vi "SR830_Keithley_Data_Recorder.vi"() -> ()   [LabVIEW 2021]
uses:
  <instrlib>/Stanford Research 830/Stanford Research 830.lvlib
  <instrlib>/Stanford Research 830/Public/Data/Read (All Parameters).vi
panel:
  out "current time":timestamp
  out "X-Value 3":dbl
  out "Theta-Value 3":dbl
  out "R-Value 3":dbl
  in  "System #3 Enabled/Disabled":bool
  in  "SR830 #3":refnum<visa-resource-name>="GPIB0::10::INSTR"
  in  "SR830 #3 Input Connection":u16(ring) items=["Single-Ended Voltage", "Differential Voltage", "1 MOhm Current Gain", "100 MOhm Current Gain"]
  in  "SR830 #3\nInput Coupling":u16(ring) items=["AC", "DC"]
  in  "SR830 #3 Input \nShield Grounding":u16(ring) items=["Float", "Ground"]
  in  "SR830 #3 Input\nNotch Filter":u16(ring) items=["None", "Line Notch", "2x Line Notch", "Both Notch Filters"]
  in  "SR830 #3 Trigger Source":u16(ring) items=["Internal", "External"]
  in  "SR830 #3 Internal \nReference Frequency":dbl=17.0
  in  "SR830 #3 Detection Harm. Num.":dbl=1.0
  in  "SR830 #3 Sine \nOutput Amplitude":dbl=1.0
  in  "SR830 #3 Reference Source":u16(ring)=1 items=["External", "Internal"]
  in  "SR830 #3 Manual \nPhase":dbl
  in  "SR830 #3 \nAuto Phase":bool
  in  "SR830 #3 \nTime Constant":u16(ring)=9 items=["10 us", "30 us", "100 us", "300 us", "1 ms", "3 ms", "10 ms", "30 ms", "100 ms", "300 ms", "1 s", "3 s", "10 s", "30 s", "100 s", "300 s", "1 ks", "3 ks", "10 ks", "30 ks"]
  in  "SR830 #3 Low\nPass Filter Slope":u16(ring)=3 items=["6 dB/oct", "12 dB/oct", "18 db/oct", "24 dB/oct"]
  in  "SR830 #3\nSync Filter":bool
  in  "SR830 #3 \nDynamic Reserve":i16(ring)=1 items=["Auto Reserve"=-1, "High Reserve"=0, "Normal"=1, "Low Noise"=2]
  in  "SR830 #3\nSensitivity":i16(ring)=17 items=["Auto Gain"=-1, "2 nV/fA"=0, "5 nV/fA"=1, "10 nV/fA"=2, "20 nV/fA"=3, "50 nV/fA"=4, "100 nV/fA"=5, "200 nV/fA"=6, "500 nV/fA"=7, "1 uV/pA"=8, "2 uV/pA"=9, "5 uV/pA"=10, "10 uV/pA"=11, "20 uV/pA"=12, "50 uV/pA"=13, "100 uV/pA"=14, "200 uV/pA"=15, "500 uV/pA"=16, "1 mV/nA"=17, "2 mV/nA"=18, "5 mV/nA"=19, "10 mV/nA"=20, "20 mV/nA"=21, "50 mV/nA"=22, "100 mV/nA"=23, "200 mV/nA"=24, "500 mV/mA"=25, "1 V/uA"=26]
  out "X-Value 2":dbl
  out "Theta-Value 2":dbl
  out "R-Value 2":dbl
  in  "System #2 Enabled/Disabled":bool
  in  "SR830 #2":refnum<visa-resource-name>="GPIB0::10::INSTR"
  in  "SR830 #2 Input Connection":u16(ring) items=["Single-Ended Voltage", "Differential Voltage", "1 MOhm Current Gain", "100 MOhm Current Gain"]
  in  "SR830 #2\nInput Coupling":u16(ring) items=["AC", "DC"]
  in  "SR830 #2 Input \nShield Grounding":u16(ring) items=["Float", "Ground"]
  in  "SR830 #2 Input\nNotch Filter":u16(ring) items=["None", "Line Notch", "2x Line Notch", "Both Notch Filters"]
  in  "SR830 #2 Trigger Source":u16(ring) items=["Internal", "External"]
  in  "SR830 #2 Internal \nReference Frequency":dbl=17.0
  in  "SR830 #2 Detection Harm. Num.":dbl=1.0
  in  "SR830 #2 Sine \nOutput Amplitude":dbl=1.0
  in  "SR830 #2 Reference Source":u16(ring)=1 items=["External", "Internal"]
  in  "SR830 #2 Manual \nPhase":dbl
  in  "SR830 #2 \nAuto Phase":bool
  in  "SR830 #2 \nTime Constant":u16(ring)=9 items=["10 us", "30 us", "100 us", "300 us", "1 ms", "3 ms", "10 ms", "30 ms", "100 ms", "300 ms", "1 s", "3 s", "10 s", "30 s", "100 s", "300 s", "1 ks", "3 ks", "10 ks", "30 ks"]
  in  "SR830 #2 Low\nPass Filter Slope":u16(ring)=3 items=["6 dB/oct", "12 dB/oct", "18 db/oct", "24 dB/oct"]
  in  "SR830 #2\nSync Filter":bool
  in  "SR830 #2 \nDynamic Reserve":i16(ring)=1 items=["Auto Reserve"=-1, "High Reserve"=0, "Normal"=1, "Low Noise"=2]
  in  "SR830 #2\nSensitivity":i16(ring)=17 items=["Auto Gain"=-1, "2 nV/fA"=0, "5 nV/fA"=1, "10 nV/fA"=2, "20 nV/fA"=3, "50 nV/fA"=4, "100 nV/fA"=5, "200 nV/fA"=6, "500 nV/fA"=7, "1 uV/pA"=8, "2 uV/pA"=9, "5 uV/pA"=10, "10 uV/pA"=11, "20 uV/pA"=12, "50 uV/pA"=13, "100 uV/pA"=14, "200 uV/pA"=15, "500 uV/pA"=16, "1 mV/nA"=17, "2 mV/nA"=18, "5 mV/nA"=19, "10 mV/nA"=20, "20 mV/nA"=21, "50 mV/nA"=22, "100 mV/nA"=23, "200 mV/nA"=24, "500 mV/mA"=25, "1 V/uA"=26]
  out "R-Value":dbl
  out "Theta-Value":dbl
  out "X-Value":dbl
  in  "SR830 #1\nSensitivity":i16(ring)=17 items=["Auto Gain"=-1, "2 nV/fA"=0, "5 nV/fA"=1, "10 nV/fA"=2, "20 nV/fA"=3, "50 nV/fA"=4, "100 nV/fA"=5, "200 nV/fA"=6, "500 nV/fA"=7, "1 uV/pA"=8, "2 uV/pA"=9, "5 uV/pA"=10, "10 uV/pA"=11, "20 uV/pA"=12, "50 uV/pA"=13, "100 uV/pA"=14, "200 uV/pA"=15, "500 uV/pA"=16, "1 mV/nA"=17, "2 mV/nA"=18, "5 mV/nA"=19, "10 mV/nA"=20, "20 mV/nA"=21, "50 mV/nA"=22, "100 mV/nA"=23, "200 mV/nA"=24, "500 mV/mA"=25, "1 V/uA"=26]
  in  "SR830 #1 \nDynamic Reserve":i16(ring)=1 items=["Auto Reserve"=-1, "High Reserve"=0, "Normal"=1, "Low Noise"=2]
  in  "SR830 #1\nSync Filter":bool
  in  "SR830 #1 Low\nPass Filter Slope":u16(ring)=3 items=["6 dB/oct", "12 dB/oct", "18 db/oct", "24 dB/oct"]
  in  "SR830 #1 \nTime Constant":u16(ring)=8 items=["10 us", "30 us", "100 us", "300 us", "1 ms", "3 ms", "10 ms", "30 ms", "100 ms", "300 ms", "1 s", "3 s", "10 s", "30 s", "100 s", "300 s", "1 ks", "3 ks", "10 ks", "30 ks"]
  in  "SR830 #1 \nAuto Phase":bool
  in  "SR830 #1 Manual \nPhase":dbl
  in  "SR830 #1 Reference Source":u16(ring)=1 items=["External", "Internal"]
  in  "SR830 #1 Sine \nOutput Amplitude":dbl=1.0
  in  "SR830 #1 Detection Harm. Num.":dbl=1.0
  in  "SR830 #1 Internal \nReference Frequency":dbl=17.0
  in  "SR830 #1 Trigger Source":u16(ring) items=["Internal", "External"]
  in  "SR830 #1 Input\nNotch Filter":u16(ring) items=["None", "Line Notch", "2x Line Notch", "Both Notch Filters"]
  in  "SR830 #1 Input \nShield Grounding":u16(ring) items=["Float", "Ground"]
  in  "SR830 #1\nInput Coupling":u16(ring) items=["AC", "DC"]
  in  "SR830 #1 Input Connection":u16(ring) items=["Single-Ended Voltage", "Differential Voltage", "1 MOhm Current Gain", "100 MOhm Current Gain"]
  in  "SR830 #1":refnum<visa-resource-name>="GPIB0::10::INSTR"
  in  "System #1 Enabled/Disabled":bool
  in  "System Reset All?":bool
  in  "program_stop":bool
  out "Actual Save Path":path
  in  "<File Name>.txt (Don't add extension)":string
  in  "Data Save Path:":path=path "C:/Users/labpc/Documents/ProbeStation Users Data"
  # "SR830"
  # "SR830"
  # "SR830"
  # "Input Signal"
  # "Input Signal"
  # "Input Signal"
  # "Readout (Recorded)"
  # "Readout (Recorded)"
  # "Readout (Recorded)"
  # "Source / Reference"
  # "Source / Reference"
  # "Source / Reference"
  # "Input Filters & Sens"
  # "Input Filters & Sens"
  # "Input Filters & Sens"
  # "Initialisation:\n--> Reset \n--> Instruments?"
  # "File I/O"
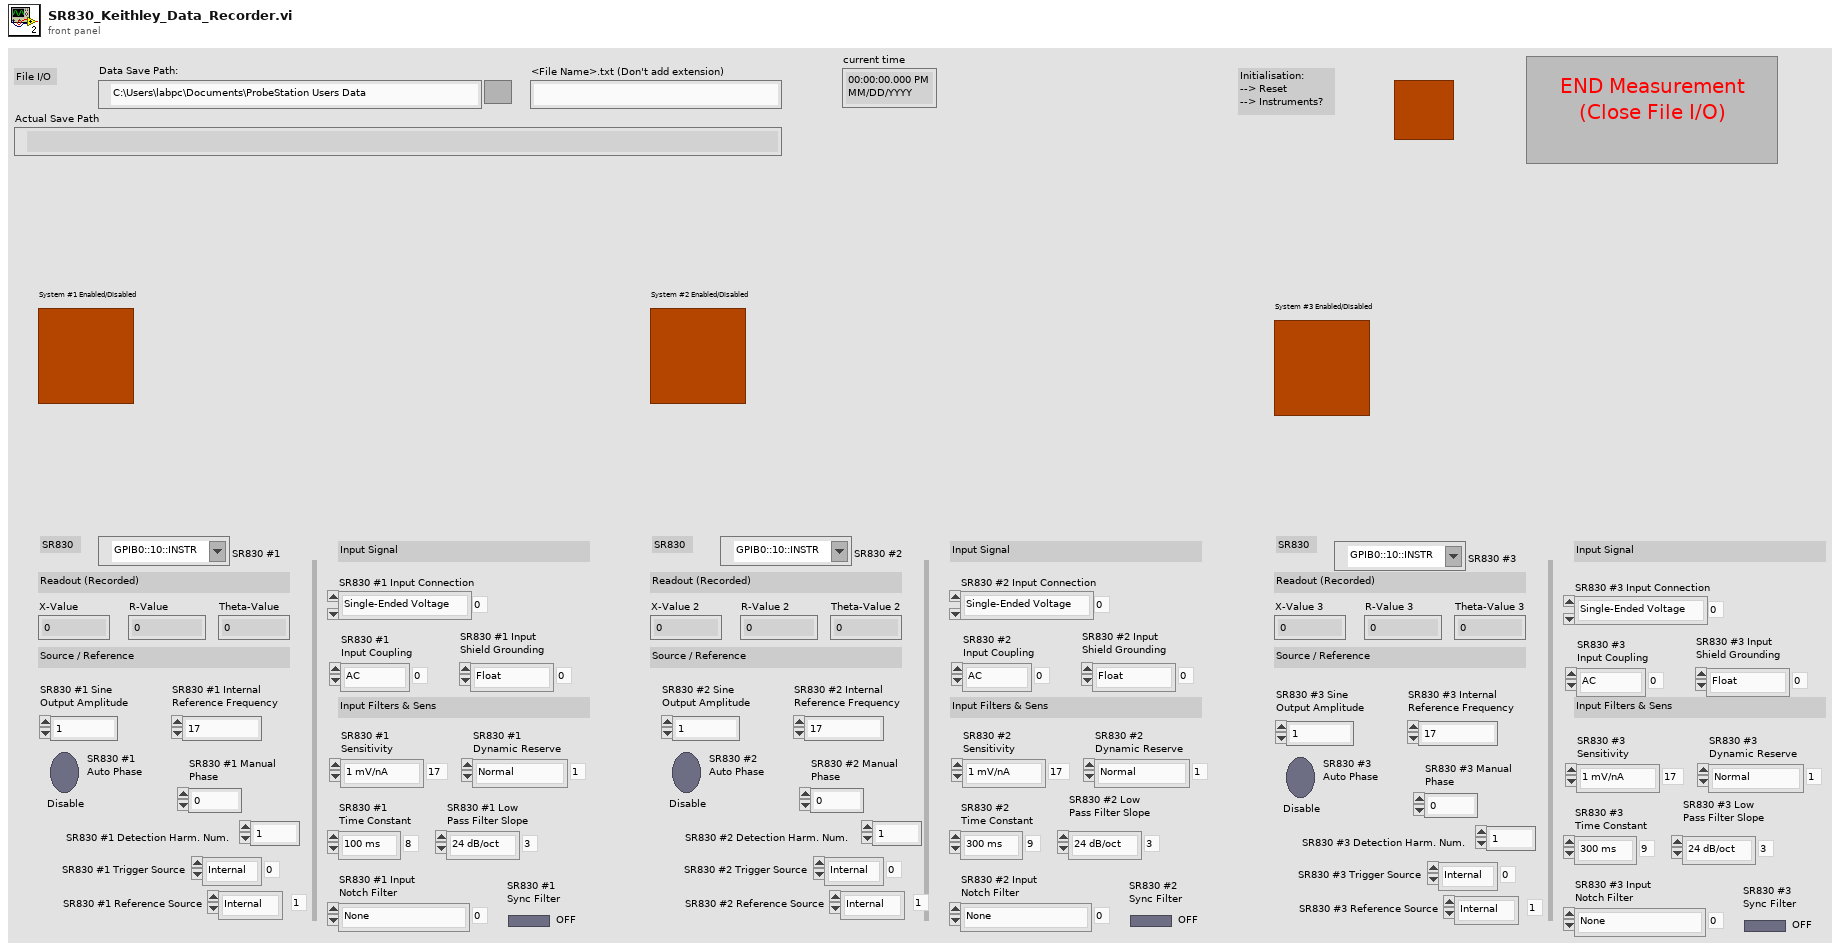
[diagram p1: front panel]
types:
  T1 = enum16{"open", "replace", "create", "open or create", "replace or create", "replace or create with confirmation"}
  T2 = cluster{"VISA resource name out":refnum<visa-resource-name>, "error out":errorcluster}
  T3 = cluster{"array":dbl[][], "array":dbl[][], "array":dbl[][]}
  T4 = cluster{"System #1 Enabled/Disabled":bool, "System #2 Enabled/Disabled":bool, "System #3 Enabled/Disabled":bool}
  T5 = cluster{"Voltage":sgl, "Current":sgl, "X-Value":dbl}
  T6 = cluster{"X-Value":dbl, "Y-Value":dbl, "R-Value":dbl, "Theta-Value":dbl, "Aux In 1 Value":dbl, "Aux In 2 Value":dbl, "Aux In 3 Value":dbl, "Aux In 4 Value":dbl, "Reference Frequency":dbl, "Channel 1 Display":dbl, "Channel 2 Display":dbl}
  T7 = cluster{"X-Value":dbl, "R-Value":dbl, "Theta-Value":dbl}
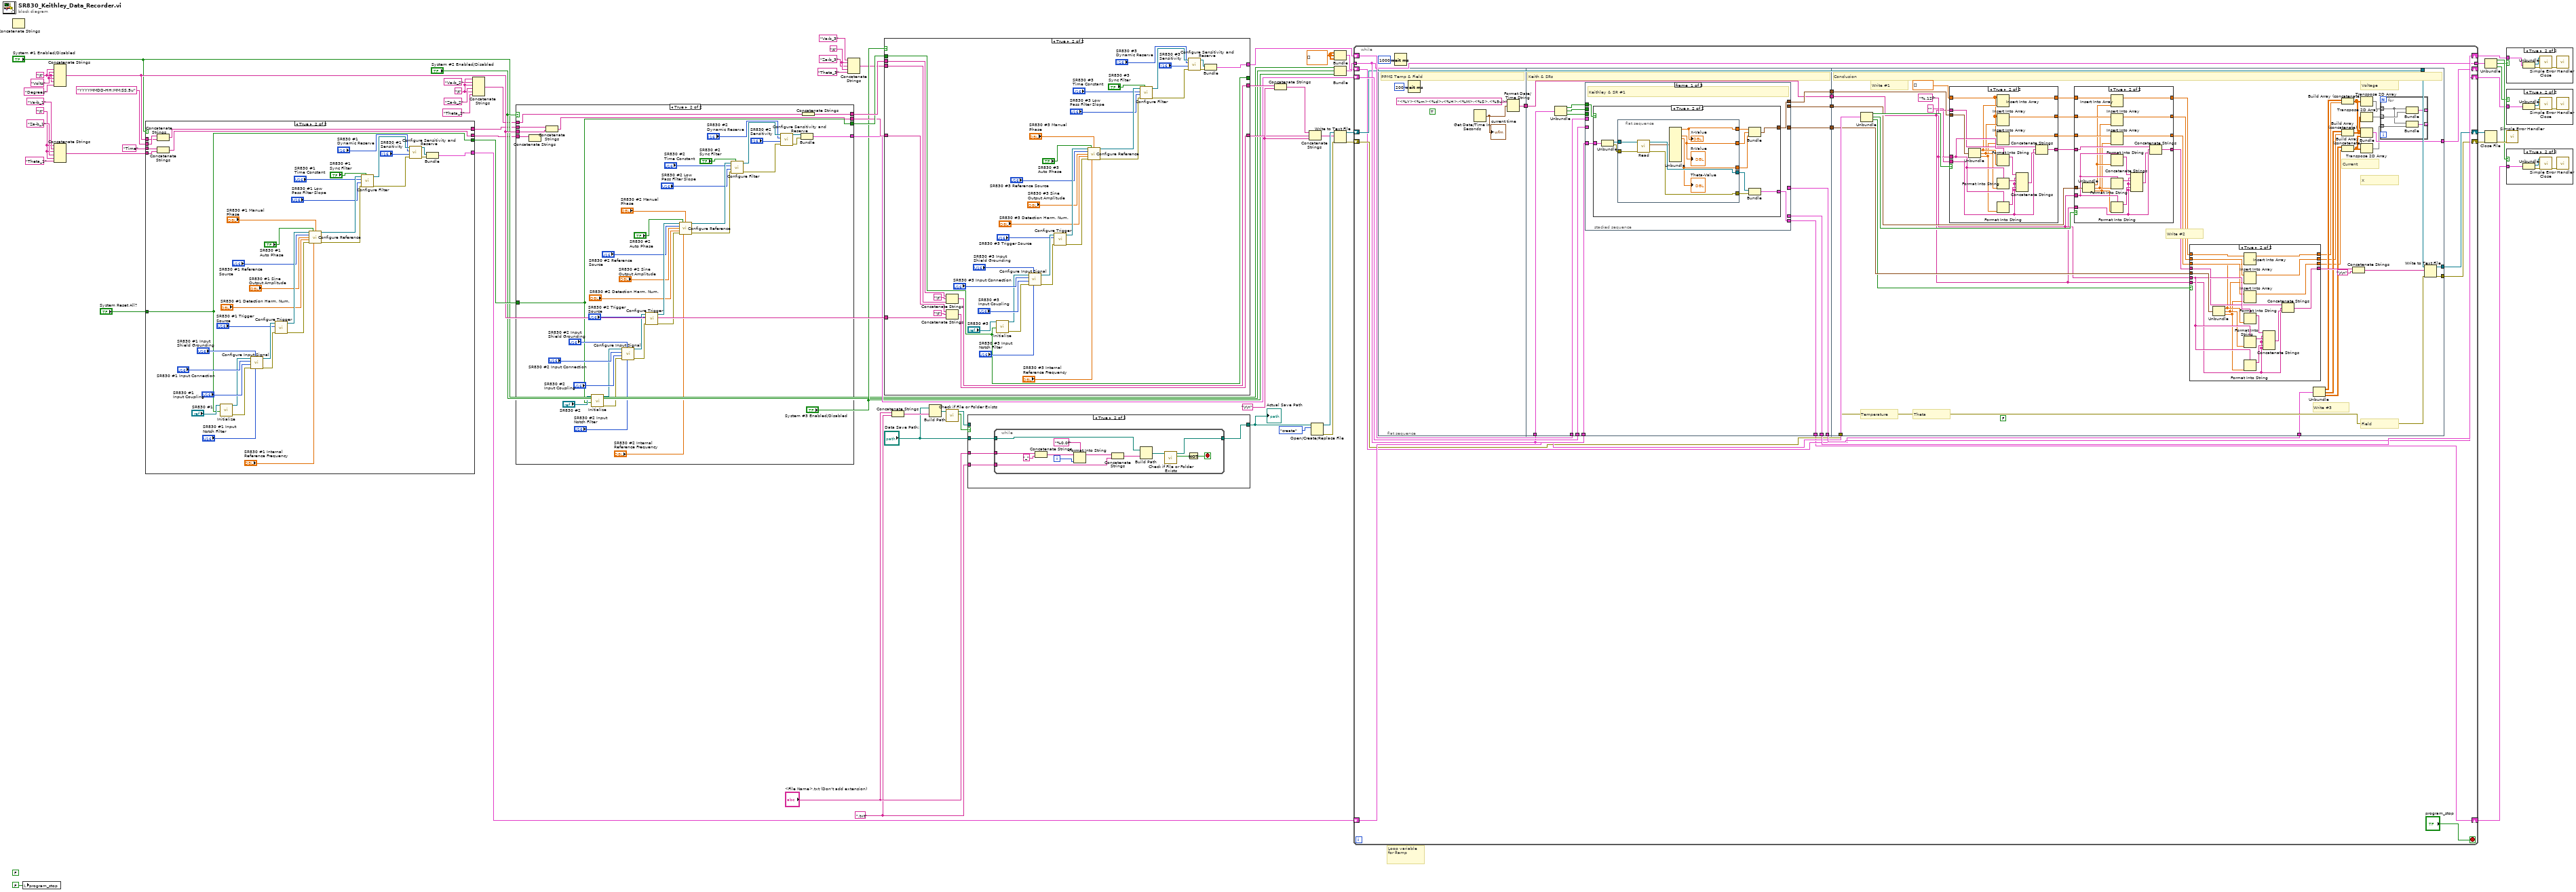
[diagram p0: block diagram]
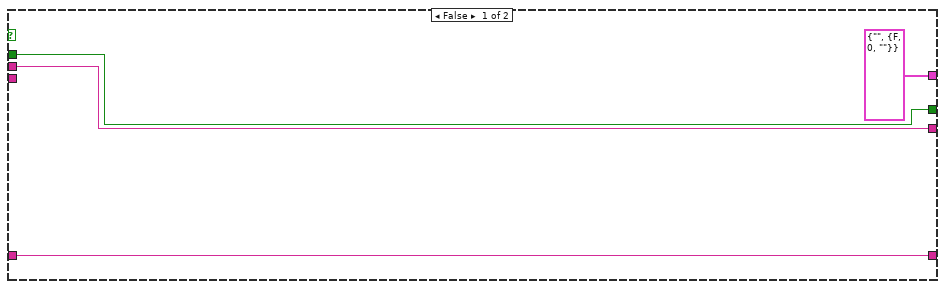
[diagram p5: hidden frame]
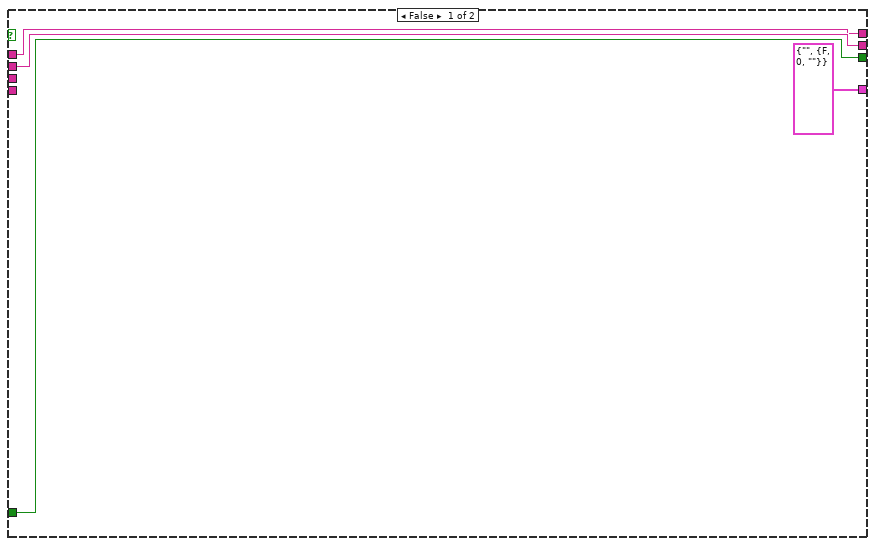
[diagram p6: hidden frame]
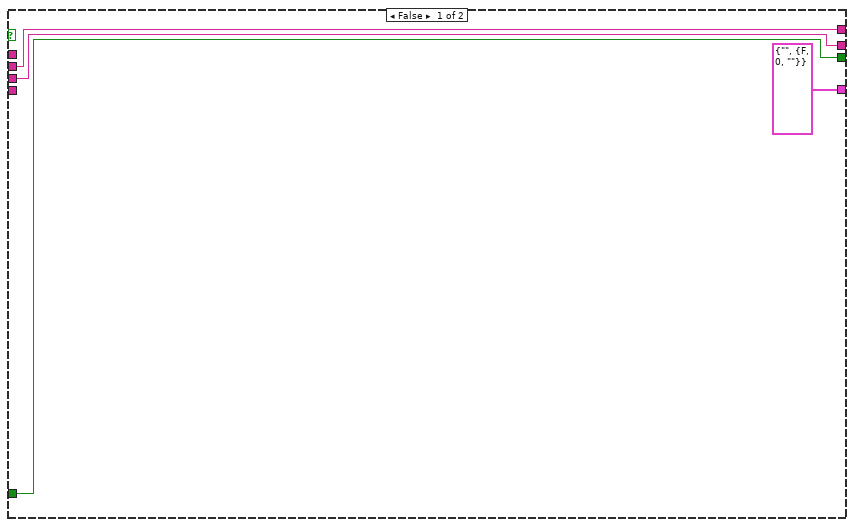
[diagram p7: hidden frame]
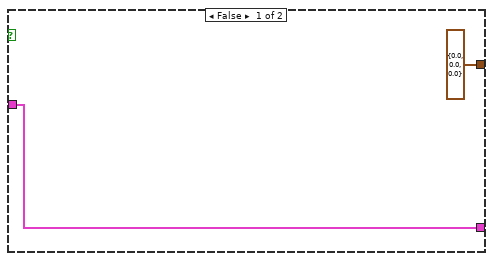
[diagram p9: hidden frame]
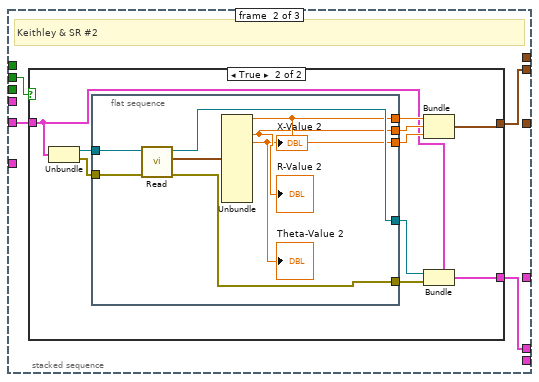
[diagram p10: hidden frame]
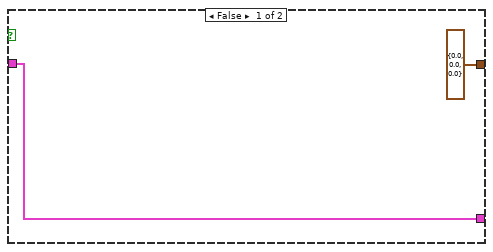
[diagram p11: hidden frame]
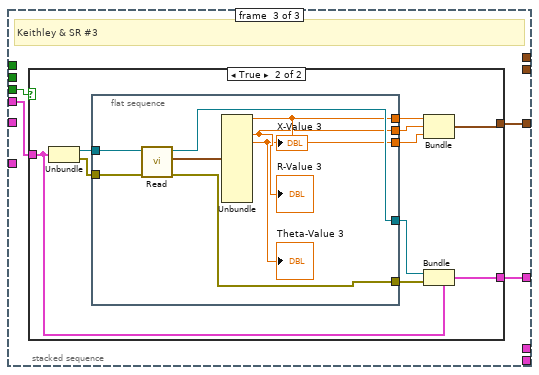
[diagram p12: hidden frame]
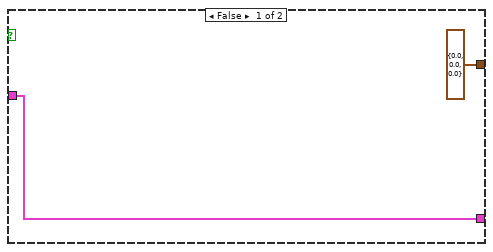
[diagram p13: hidden frame]
diagram:
  w15 = "\t"
  w3 = "\t"
  w26 = dbl[][] [] ("array")
  w4 = "\t"
  w6 = "Volts" ("string")
  w47 = "\r\n"
  w8 = "\t"
  w60 = ".txt"
  (unwired) FALSE ("Measuring")
  # "Loop variable \nfor Ramp"
  n1 = Concatenate Strings() -> ()  [unwired: 3 in, 1 out]
  n2 = local write "program_stop"(FALSE ("program_stop")) -> ()
  n3 = Concatenate Strings(w4, w6, w4, w6, w4, "Degrees" ("string")) -> (w50:string)  [unwired: 1 in]
  n4 = Concatenate Strings(w8, "Va-b_1" ("string"), w8, "Za-b_1" ("string"), w8, "Theta_1" ("string")) -> (w54:string)
  n5 = case shown="True" "System #1 Enabled/Disabled" {
    tunnel: w54 -> [_ w73]
    tunnel: "System Reset All?" -> [w70 w80]
    tunnel: [w70 w80] -> w56
    tunnel: [w68 w79] -> w2
    tunnel: w50 -> [_ w72]
    tunnel: [T2 {"VISA resource name out"="", "error out"={"status"=FALSE, "code"=0, "source"=""}} w76] -> w39
    tunnel: "Time" ("string") -> [w68 w75]
    tunnel: "YYYYMMDD-HH:MM:SS.5u" ("string") -> [w67 w74]
    tunnel: [w67 w71] -> w1
    frame False {
    }
    frame True {
      n6 = Concatenate Strings(w74, w72) -> (w71:string)
      n7 = Concatenate Strings(w75, w73) -> (w79:string)
      n8 = call <instrlib>:"Initialize.vi"("Reset (True)"=w80, "VISA resource name"="SR830 #1") -> ("error out"=w103:errorcluster, "VISA resource name out"=w104:refnum<visa-resource-name>)  [unwired: 8 in]
      n9 = call <instrlib>:"Configure Input Signal.vi"("Input Notch Filter (0: None)"="SR830 #1 Input\nNotch Filter", "Input Shield Grounding (0: Float)"="SR830 #1 Input \nShield Grounding", "error in (no error)"=w103, "Input Coupling (0: AC)"="SR830 #1\nInput Coupling", "Input Connection (0: Single-Ended Voltage)"="SR830 #1 Input Connection", "VISA resource name"=w104) -> ("error out"=w101:errorcluster, "VISA resource name out"=w102:refnum<visa-resource-name>)  [unwired: 4 in]
      n10 = call <instrlib>:"Configure Trigger.vi"("error in (no error)"=w101, "Trigger Source (0: Internal)"="SR830 #1 Trigger Source", "VISA resource name"=w102) -> ("error out"=w99:errorcluster, "VISA resource name out"=w100:refnum<visa-resource-name>)  [unwired: 7 in]
      n11 = call <instrlib>:"Configure Reference.vi"("VISA resource name"=w100, "Auto Phase (T: Enabled)"="SR830 #1 \nAuto Phase", "Manual Phase (0 Degree)"="SR830 #1 Manual \nPhase", "Reference Source (1: Internal)"="SR830 #1 Reference Source", "Sine Output Amplitude (1 V)"="SR830 #1 Sine \nOutput Amplitude", "Detection Harmonic Number (1)"="SR830 #1 Detection Harm. Num.", "error in (no error)"=w99, "Internal Reference Frequency (1000 Hz)"="SR830 #1 Internal \nReference Frequency") -> ("VISA resource name out"=w97:refnum<visa-resource-name>, "error out"=w98:errorcluster)  [unwired: 6 in]
      n12 = call <instrlib>:"Configure Filter.vi"("Enable Sync Filter (F: Disable)"="SR830 #1\nSync Filter", "error in (no error)"=w98, "Low Pass Filter Slope (1: 12dB/oct)"="SR830 #1 Low\nPass Filter Slope", "Time Constant (8: 100ms)"="SR830 #1 \nTime Constant", "VISA resource name"=w97) -> ("error out"=w83:errorcluster, "VISA resource name out"=w84:refnum<visa-resource-name>)  [unwired: 5 in]
      n13 = call <instrlib>:"Configure Sensitivity and Reserve.vi"("error in (no error)"=w83, "Sensitivity (-1: Auto gain)"="SR830 #1\nSensitivity", "Dynamic Reserve (-1: Auto Reserve)"="SR830 #1 \nDynamic Reserve", "VISA resource name"=w84) -> ("error out"=w77:errorcluster, "VISA resource name out"=w78:refnum<visa-resource-name>)  [unwired: 6 in]
      n14 = Bundle("VISA resource name out"=w78, "error out"=w77) -> (w76:T2)  [unwired: 1 in]
    }
  }
  n15 = Concatenate Strings(w3, "Va-b_2" ("string"), w3, "Za-b_2" ("string"), w3, "Theta_2" ("string")) -> (w11:string)
  n16 = case shown="True" "System #2 Enabled/Disabled" {
    tunnel: w11 -> [w108 w148]
    tunnel: [w108 w147] -> w55
    tunnel: w56 -> [w111 w119]
    tunnel: [w111 w119] -> w53
    tunnel: w1 -> [w110 w118]
    tunnel: [w110 w117] -> w51
    tunnel: w50 -> [_ w112]
    tunnel: [T2 {"VISA resource name out"="", "error out"={"status"=FALSE, "code"=0, "source"=""}} w114] -> w38
    tunnel: w2 -> [_ w113]
    frame False {
    }
    frame True {
      n17 = Concatenate Strings(w113) -> ()  [unwired: 1 in, 1 out]
      n18 = Concatenate Strings(w118, w112) -> (w117:string)
      n19 = call <instrlib>:"Initialize.vi"("Reset (True)"=w119, "VISA resource name"="SR830 #2") -> ("error out"=w142:errorcluster, "VISA resource name out"=w143:refnum<visa-resource-name>)  [unwired: 8 in]
      n20 = call <instrlib>:"Configure Input Signal.vi"("Input Notch Filter (0: None)"="SR830 #2 Input\nNotch Filter", "Input Shield Grounding (0: Float)"="SR830 #2 Input \nShield Grounding", "error in (no error)"=w142, "Input Coupling (0: AC)"="SR830 #2\nInput Coupling", "Input Connection (0: Single-Ended Voltage)"="SR830 #2 Input Connection", "VISA resource name"=w143) -> ("error out"=w140:errorcluster, "VISA resource name out"=w141:refnum<visa-resource-name>)  [unwired: 4 in]
      n21 = call <instrlib>:"Configure Trigger.vi"("error in (no error)"=w140, "Trigger Source (0: Internal)"="SR830 #2 Trigger Source", "VISA resource name"=w141) -> ("error out"=w138:errorcluster, "VISA resource name out"=w139:refnum<visa-resource-name>)  [unwired: 7 in]
      n22 = call <instrlib>:"Configure Reference.vi"("VISA resource name"=w139, "Auto Phase (T: Enabled)"="SR830 #2 \nAuto Phase", "Manual Phase (0 Degree)"="SR830 #2 Manual \nPhase", "Reference Source (1: Internal)"="SR830 #2 Reference Source", "Sine Output Amplitude (1 V)"="SR830 #2 Sine \nOutput Amplitude", "Detection Harmonic Number (1)"="SR830 #2 Detection Harm. Num.", "error in (no error)"=w138, "Internal Reference Frequency (1000 Hz)"="SR830 #2 Internal \nReference Frequency") -> ("VISA resource name out"=w136:refnum<visa-resource-name>, "error out"=w137:errorcluster)  [unwired: 6 in]
      n23 = call <instrlib>:"Configure Filter.vi"("Enable Sync Filter (F: Disable)"="SR830 #2\nSync Filter", "error in (no error)"=w137, "Low Pass Filter Slope (1: 12dB/oct)"="SR830 #2 Low\nPass Filter Slope", "Time Constant (8: 100ms)"="SR830 #2 \nTime Constant", "VISA resource name"=w136) -> ("error out"=w122:errorcluster, "VISA resource name out"=w123:refnum<visa-resource-name>)  [unwired: 5 in]
      n24 = call <instrlib>:"Configure Sensitivity and Reserve.vi"("error in (no error)"=w122, "Sensitivity (-1: Auto gain)"="SR830 #2\nSensitivity", "Dynamic Reserve (-1: Auto Reserve)"="SR830 #2 \nDynamic Reserve", "VISA resource name"=w123) -> ("error out"=w115:errorcluster, "VISA resource name out"=w116:refnum<visa-resource-name>)  [unwired: 6 in]
      n25 = Bundle("VISA resource name out"=w116, "error out"=w115) -> (w114:T2)  [unwired: 1 in]
      n26 = Concatenate Strings(w148) -> (w147:string)
    }
  }
  n27 = Concatenate Strings("Va-b_3" ("string"), w15, "Za-b_3" ("string"), w15, "Theta_3" ("string")) -> (w10:string)
  n28 = case shown="True" "System #3 Enabled/Disabled" {
    tunnel: w10 -> [_ w191]
    tunnel: w55 -> [w152 w189]
    tunnel: [w152 w188] -> w52
    tunnel: w53 -> [w151 w160]
    tunnel: [w151 w160] -> _
    tunnel: w51 -> [w150 w158]
    tunnel: w50 -> [_ w157]
    tunnel: [w150 w156] -> w45
    tunnel: [T2 {"VISA resource name out"="", "error out"={"status"=FALSE, "code"=0, "source"=""}} w153] -> w37
    frame False {
    }
    frame True {
      n29 = Concatenate Strings(w189, "\t", w191) -> (w188:string)
      n30 = Concatenate Strings(w158, "\t", w157) -> (w156:string)
      n31 = call <instrlib>:"Initialize.vi"("Reset (True)"=w160, "VISA resource name"="SR830 #3") -> ("error out"=w183:errorcluster, "VISA resource name out"=w184:refnum<visa-resource-name>)  [unwired: 8 in]
      n32 = call <instrlib>:"Configure Input Signal.vi"("Input Notch Filter (0: None)"="SR830 #3 Input\nNotch Filter", "Input Shield Grounding (0: Float)"="SR830 #3 Input \nShield Grounding", "error in (no error)"=w183, "Input Coupling (0: AC)"="SR830 #3\nInput Coupling", "Input Connection (0: Single-Ended Voltage)"="SR830 #3 Input Connection", "VISA resource name"=w184) -> ("error out"=w181:errorcluster, "VISA resource name out"=w182:refnum<visa-resource-name>)  [unwired: 4 in]
      n33 = call <instrlib>:"Configure Trigger.vi"("error in (no error)"=w181, "Trigger Source (0: Internal)"="SR830 #3 Trigger Source", "VISA resource name"=w182) -> ("error out"=w179:errorcluster, "VISA resource name out"=w180:refnum<visa-resource-name>)  [unwired: 7 in]
      n34 = call <instrlib>:"Configure Reference.vi"("VISA resource name"=w180, "Auto Phase (T: Enabled)"="SR830 #3 \nAuto Phase", "Manual Phase (0 Degree)"="SR830 #3 Manual \nPhase", "Reference Source (1: Internal)"="SR830 #3 Reference Source", "Sine Output Amplitude (1 V)"="SR830 #3 Sine \nOutput Amplitude", "Detection Harmonic Number (1)"="SR830 #3 Detection Harm. Num.", "error in (no error)"=w179, "Internal Reference Frequency (1000 Hz)"="SR830 #3 Internal \nReference Frequency") -> ("VISA resource name out"=w177:refnum<visa-resource-name>, "error out"=w178:errorcluster)  [unwired: 6 in]
      n35 = call <instrlib>:"Configure Filter.vi"("Enable Sync Filter (F: Disable)"="SR830 #3\nSync Filter", "error in (no error)"=w178, "Low Pass Filter Slope (1: 12dB/oct)"="SR830 #3 Low\nPass Filter Slope", "Time Constant (8: 100ms)"="SR830 #3 \nTime Constant", "VISA resource name"=w177) -> ("error out"=w163:errorcluster, "VISA resource name out"=w164:refnum<visa-resource-name>)  [unwired: 5 in]
      n36 = call <instrlib>:"Configure Sensitivity and Reserve.vi"("error in (no error)"=w163, "Sensitivity (-1: Auto gain)"="SR830 #3\nSensitivity", "Dynamic Reserve (-1: Auto Reserve)"="SR830 #3 \nDynamic Reserve", "VISA resource name"=w164) -> ("error out"=w154:errorcluster, "VISA resource name out"=w155:refnum<visa-resource-name>)  [unwired: 6 in]
      n37 = Bundle("VISA resource name out"=w155, "error out"=w154) -> (w153:T2)  [unwired: 1 in]
    }
  }
  n38 = Concatenate Strings("<File Name>.txt (Don't add extension)", w60) -> (w66:string)
  n39 = Build Path(base path="Data Save Path:", name or relative path=w66) -> (appended path=w65:path)
  n40 = call <vilib>:"Check if File or Folder Exists.vi"("path"=w65) -> ("file or folder exists?"=w64:bool, "dup path"=w63:path)  [unwired: 8 in, 1 out]
  n41 = case shown="True" w64 {
    tunnel: [w192 w193] -> w58
    tunnel: w63 -> [w192 _]
    tunnel: "Data Save Path:" -> [_ w194]
    tunnel: "<File Name>.txt (Don't add extension)" -> [_ w196]
    tunnel: w60 -> [_ w195]
    frame False {
    }
    frame True {
      n42 = while {
        tunnel: w196 -> [w199]
        tunnel: w195 -> [w204]
        tunnel: w194 -> [w202]
        tunnel: [w200] -> w193
        i -> [w206]
        stop <- w208 stop-if-true
        n43 = Concatenate Strings(w199, "_" ("string")) -> (w198:string)
        n44 = Format Into String(format string="%0.0f", initial string=w198, w206) -> (resulting string=w205:string)  [unwired: 1 in, 1 out]
        n45 = Concatenate Strings(w205, w204) -> (w203:string)
        n46 = Build Path(base path=w202, name or relative path=w203) -> (appended path=w201:path)
        n47 = call <vilib>:"Check if File or Folder Exists.vi"("path"=w201) -> ("file or folder exists?"=w209:bool, "dup path"=w200:path)  [unwired: 8 in, 1 out]
        n48 = Not(x=w209) -> (.not. x?=w208:bool)
      }
    }
  }
  "Actual Save Path" <- w58
  n49 = Concatenate Strings(w52, w47) -> (w46:string)
  n50 = Concatenate Strings(w46, w45, w47) -> (w44:string)
  n51 = Open/Create/Replace File(file path (use dialog)=w58, operation (0:open)=T1."create") -> (refnum out=w49:refnum<file>, error out=w48:errorcluster)  [unwired: 4 in, 1 out]
  n52 = Bundle("array"=w26, "array"=w26, "array"=w26) -> (w27:T3)  [unwired: 1 in]
  n53 = Bundle("System #1 Enabled/Disabled"="System #1 Enabled/Disabled", "System #2 Enabled/Disabled"="System #2 Enabled/Disabled", "System #3 Enabled/Disabled"="System #3 Enabled/Disabled") -> (w33:T4)  [unwired: 1 in]
  n54 = Write to Text File(file (use dialog)=w49, text=w44, error in=w48) -> (refnum out=w28:refnum<file>, error out=w42:errorcluster)  [unwired: 1 in, 1 out]
  n55 = while {
    shift-right: [w217] -> w41
    shift-left: w28 -> [w218]
    shift-right: [w215] -> w40
    shift-left: w42 -> [w216]
    shift-right: [w213] -> w25
    shift-left: w39 -> [w227]
    shift-right: [w224] -> w23
    shift-left: w38 -> [w226]
    shift-right: [w223] -> w24
    shift-left: w37 -> [w225]
    tunnel: w33 -> [w219]
    tunnel: [w219] -> w32
    shift-right: [w212] -> _
    shift-left: w27 -> [w214]
    stop <- "program_stop" stop-if-true
    n56 = flat-sequence {
      tunnel: [w230] -> w211
      tunnel: w227 -> [w238]
      tunnel: w226 -> [w247]
      tunnel: w225 -> [w246]
      tunnel: [w236] -> w224
      tunnel: [w235] -> w223
      tunnel: w219 -> [w245]
      tunnel: [w241] -> w222
      tunnel: [w240] -> w221
      tunnel: [w239] -> w220
      tunnel: [w237] -> w213
      tunnel: w211 -> [w234]
      tunnel: [w234] -> w210
      tunnel: w222 -> [w357]
      tunnel: w221 -> [w356]
      tunnel: w220 -> [w355]
      tunnel: w219 -> [w359]
      tunnel: w218 -> [w346]
      tunnel: w216 -> [w344]
      tunnel: [w345] -> w217
      tunnel: [w343] -> w215
      tunnel: w214 -> [w339]
      tunnel: [w338] -> w212
      tunnel: w210 -> [w321]
      frame #0 {
        (unwired) TRUE ("Measuring")
        # "PPMS Temp & Field"
        n57 = Wait (ms)(milliseconds to wait=u32 200) -> ()  [unwired: 1 out]
        n58 = Get Date/Time In Seconds() -> (seconds since 1Jan1904=w232:timestamp)
        "current time" <- w232
        n59 = Format Date/Time String(time format string (%c)="<%Y><%m><%d>-<%H>:<%M>:<%S>.<%5u>" ("string"), seconds (now)=w232) -> (date/time string=w230:string)  [unwired: 1 in]
      }
      frame #1 {
        # "Keith & SRs"
        n60 = Unbundle(w245) -> ("System #1 Enabled/Disabled"=w244:bool, "System #2 Enabled/Disabled"=w243:bool, "System #3 Enabled/Disabled"=w242:bool)
        n61 = stacked-sequence {
          tunnel: w247 -> [_ w275 _]
          tunnel: w246 -> [_ _ w299]
          tunnel: [w248 _ _] -> w237
          tunnel: [_ w272 _] -> w236
          tunnel: w244 -> [w251 _ _]
          tunnel: w243 -> [_ w274 _]
          tunnel: w242 -> [_ _ w298]
          tunnel: [w250 _ _] -> w241
          tunnel: [_ w273 _] -> w240
          tunnel: [_ _ w297] -> w239
          tunnel: w238 -> [w249 _ _]
          tunnel: [_ _ w296] -> w235
          frame #0 {
            # "Keithley & SR #1"
            n62 = case shown="True" w251 {
              tunnel: [w252 w263] -> w248
              tunnel: [T5 {"Voltage"=0.0, "Current"=0.0, "X-Value"=0.0} w257] -> w250
              tunnel: w249 -> [w252 w256]
              frame False {
              }
              frame True {
                n63 = Unbundle(w256) -> ("VISA resource name out"=w255:refnum<visa-resource-name>, "error out"=w254:errorcluster)
                n64 = flat-sequence {
                  tunnel: [w271] -> w262
                  tunnel: [w270] -> w261
                  tunnel: [w268] -> w260
                  tunnel: [w267] -> w259
                  tunnel: [w266] -> w258
                  tunnel: w255 -> [w265]
                  tunnel: w254 -> [w264]
                  frame #0 {
                    n65 = call-poly <instrlib>:"Read.vi"("error in (no error)"=w264, "VISA resource name"=w265) -> ("error out"=w270:errorcluster, "Parameter Values"=w269:T6, "VISA resource name out"=w271:refnum<visa-resource-name>)  [unwired: 7 in]
                    n66 = Unbundle(w269) -> ("X-Value"=w268:dbl, "R-Value"=w267:dbl, "Theta-Value"=w266:dbl)  [unwired: 8 out]
                    "X-Value" <- w268
                    "Theta-Value" <- w266
                    "R-Value" <- w267
                  }
                }
                n67 = Bundle("X-Value"=w260, "R-Value"=w259, "Theta-Value"=w258) -> (w257:T7)  [unwired: 1 in]
                n68 = Bundle("VISA resource name out"=w262, "error out"=w261) -> (w263:T2)  [unwired: 1 in]
              }
            }
          }
          frame #1 {
            # "Keithley & SR #2"
            n69 = case shown="True" w274 {
              tunnel: [w277 w287] -> w272
              tunnel: w275 -> [w277 w283]
              tunnel: [T5 {"Voltage"=0.0, "Current"=0.0, "X-Value"=0.0} w282] -> w273
              frame False {
              }
              frame True {
                n70 = Unbundle(w283) -> ("VISA resource name out"=w281:refnum<visa-resource-name>, "error out"=w280:errorcluster)
                n71 = flat-sequence {
                  tunnel: [w295] -> w279
                  tunnel: [w294] -> w278
                  tunnel: [w292] -> w286
                  tunnel: [w291] -> w285
                  tunnel: [w290] -> w284
                  tunnel: w281 -> [w289]
                  tunnel: w280 -> [w288]
                  frame #0 {
                    n72 = call-poly <instrlib>:"Read.vi"("error in (no error)"=w288, "VISA resource name"=w289) -> ("error out"=w294:errorcluster, "Parameter Values"=w293:T6, "VISA resource name out"=w295:refnum<visa-resource-name>)  [unwired: 7 in]
                    n73 = Unbundle(w293) -> ("X-Value"=w292:dbl, "R-Value"=w291:dbl, "Theta-Value"=w290:dbl)  [unwired: 8 out]
                    "X-Value 2" <- w292
                    "Theta-Value 2" <- w290
                    "R-Value 2" <- w291
                  }
                }
                n74 = Bundle("X-Value"=w286, "R-Value"=w285, "Theta-Value"=w284) -> (w282:T7)  [unwired: 1 in]
                n75 = Bundle(cluster=w283, "VISA resource name out"=w279, "error out"=w278) -> (w287:T2)
              }
            }
          }
          frame #2 {
            # "Keithley & SR #3"
            n76 = case shown="True" w298 {
              tunnel: [w301 w311] -> w296
              tunnel: w299 -> [w301 w307]
              tunnel: [T5 {"Voltage"=0.0, "Current"=0.0, "X-Value"=0.0} w306] -> w297
              frame False {
              }
              frame True {
                n77 = Unbundle(w307) -> ("VISA resource name out"=w305:refnum<visa-resource-name>, "error out"=w304:errorcluster)
                n78 = flat-sequence {
                  tunnel: [w319] -> w303
                  tunnel: [w318] -> w302
                  tunnel: [w316] -> w310
                  tunnel: [w315] -> w309
                  tunnel: [w314] -> w308
                  tunnel: w305 -> [w313]
                  tunnel: w304 -> [w312]
                  frame #0 {
                    n79 = call-poly <instrlib>:"Read.vi"("error in (no error)"=w312, "VISA resource name"=w313) -> ("error out"=w318:errorcluster, "Parameter Values"=w317:T6, "VISA resource name out"=w319:refnum<visa-resource-name>)  [unwired: 7 in]
                    n80 = Unbundle(w317) -> ("X-Value"=w316:dbl, "R-Value"=w315:dbl, "Theta-Value"=w314:dbl)  [unwired: 8 out]
                    "X-Value 3" <- w316
                    "Theta-Value 3" <- w314
                    "R-Value 3" <- w315
                  }
                }
                n81 = Bundle("X-Value"=w310, "R-Value"=w309, "Theta-Value"=w308) -> (w306:T7)  [unwired: 1 in]
                n82 = Bundle(cluster=w307, "VISA resource name out"=w303, "error out"=w302) -> (w311:T2)
              }
            }
          }
        }
      }
      frame #2 {
        w352 = "%.12f" ("format string")
        (unwired) FALSE ("Measuring")
        # "Theta"
        # "X"
        # "Current"
        # "Voltage"
        # "Field"
        # "Temperature"
        # "Write #3"
        # "Write #2"
        # "Write #1"
        # "Conclusion"
        n83 = Unbundle(w359) -> ("System #1 Enabled/Disabled"=w358:bool, "System #2 Enabled/Disabled"=w354:bool, "System #3 Enabled/Disabled"=w353:bool)
        n84 = case shown="True" w358 {
          tunnel: w357 -> [_ w426]
          tunnel: w352 -> [_ w425]
          tunnel: "" ("date/time string") -> [_ w418]
          tunnel: w321 -> [w410 w419]
          tunnel: [w410 w420] -> w351
          tunnel: dbl[] [] ("array") -> [w409 w414]
          tunnel: [w409 w413] -> w336
          tunnel: [w409 w412] -> w335
          tunnel: [w409 w411] -> w334
          frame False {
          }
          frame True {
            n85 = Unbundle(w426) -> ("X-Value"=w417:dbl, "R-Value"=w416:dbl, "Theta-Value"=w415:dbl)
            n86 = Insert Into Array(array=w414, new element=w417) -> (w413:dbl[])  [unwired: 1 in]
            n87 = Insert Into Array(array=w414, new element=w416) -> (w412:dbl[])  [unwired: 1 in]
            n88 = Insert Into Array(array=w414, new element=w415) -> (w411:dbl[])  [unwired: 1 in]
            n89 = Format Into String(format string=w425, w417) -> (resulting string=w424:string)  [unwired: 2 in, 1 out]
            n90 = Format Into String(format string=w425, w416) -> (resulting string=w423:string)  [unwired: 2 in, 1 out]
            n91 = Format Into String(format string=w425, w415) -> (resulting string=w422:string)  [unwired: 2 in, 1 out]
            n92 = Concatenate Strings(w424, w418, w423, w418, w422, w418) -> (w421:string)
            n93 = Concatenate Strings(w419, w418, w421) -> (w420:string)
          }
        }
        n94 = case shown="True" w354 {
          tunnel: w356 -> [_ w408]
          tunnel: w352 -> [_ w407]
          tunnel: w321 -> [_ w402]
          tunnel: w351 -> [w390 w403]
          tunnel: [w390 w400] -> w350
          tunnel: w336 -> [w389 w399]
          tunnel: w335 -> [w388 w398]
          tunnel: w334 -> [w387 w397]
          tunnel: [w389 w393] -> w333
          tunnel: [w388 w392] -> w332
          tunnel: [w387 w391] -> w331
          frame False {
          }
          frame True {
            n95 = Unbundle(w408) -> ("X-Value"=w396:dbl, "R-Value"=w395:dbl, "Theta-Value"=w394:dbl)
            n96 = Insert Into Array(array=w399, new element=w396) -> (w393:dbl[])  [unwired: 1 in]
            n97 = Insert Into Array(array=w398, new element=w395) -> (w392:dbl[])  [unwired: 1 in]
            n98 = Insert Into Array(array=w397, new element=w394) -> (w391:dbl[])  [unwired: 1 in]
            n99 = Format Into String(format string=w407, w396) -> (resulting string=w406:string)  [unwired: 2 in, 1 out]
            n100 = Format Into String(format string=w407, w395) -> (resulting string=w405:string)  [unwired: 2 in, 1 out]
            n101 = Format Into String(format string=w407, w394) -> (resulting string=w404:string)  [unwired: 2 in, 1 out]
            n102 = Concatenate Strings(w406, w402, w405, w402, w404, w402) -> (w401:string)
            n103 = Concatenate Strings(w403, w402, w401) -> (w400:string)
          }
        }
        n104 = case shown="True" w353 {
          tunnel: w355 -> [_ w386]
          tunnel: w352 -> [_ w385]
          tunnel: w321 -> [_ w380]
          tunnel: w350 -> [w368 w379]
          tunnel: [w368 w378] -> w349
          tunnel: w333 -> [w367 w377]
          tunnel: w332 -> [w366 w376]
          tunnel: w331 -> [w365 w375]
          tunnel: [w367 w371] -> w330
          tunnel: [w366 w370] -> w329
          tunnel: [w365 w369] -> w328
          frame False {
          }
          frame True {
            n105 = Unbundle(w386) -> ("X-Value"=w374:dbl, "R-Value"=w373:dbl, "Theta-Value"=w372:dbl)
            n106 = Insert Into Array(array=w377, new element=w374) -> (w371:dbl[])  [unwired: 1 in]
            n107 = Insert Into Array(array=w376, new element=w373) -> (w370:dbl[])  [unwired: 1 in]
            n108 = Insert Into Array(array=w375, new element=w372) -> (w369:dbl[])  [unwired: 1 in]
            n109 = Format Into String(format string=w385, w374) -> (resulting string=w384:string)  [unwired: 2 in, 1 out]
            n110 = Format Into String(format string=w385, w373) -> (resulting string=w383:string)  [unwired: 2 in, 1 out]
            n111 = Format Into String(format string=w385, w372) -> (resulting string=w382:string)  [unwired: 2 in, 1 out]
            n112 = Concatenate Strings(w384, w380, w383, w380, w382, w380) -> (w381:string)
            n113 = Concatenate Strings(w379, w380, w381) -> (w378:string)
          }
        }
        n114 = Unbundle(w339) -> ("array"=w340:dbl[][], "array"=w341:dbl[][], "array"=w342:dbl[][])
        n115 = Build Array (concatenate)(w340, w330) -> (w327:dbl[][])
        n116 = Build Array (concatenate)(w341, w329) -> (w326:dbl[][])
        n117 = Build Array (concatenate)(w342, w328) -> (w325:dbl[][])
        n118 = Concatenate Strings(w349, "\r\n") -> (w347:string)
        n119 = Transpose 2D Array(2D array=w327) -> (transposed array=w324:dbl[][])
        n120 = Transpose 2D Array(2D array=w326) -> (transposed array=w323:dbl[][])
        n121 = Bundle(w327, w326, w325) -> (w338:cluster{dbl[][], dbl[][], dbl[][]})  [unwired: 1 in]
        n122 = Transpose 2D Array(2D array=w325) -> (transposed array=w322:dbl[][])
        n123 = for {
          tunnel: w324 -> [w361] mode=indexing
          tunnel: w323 -> [w364] mode=indexing
          tunnel: [w363] -> _ mode=indexing
          tunnel: w322 -> [w360] mode=indexing
          tunnel: [w362] -> _ mode=indexing
          n124 = Bundle(w361, w364) -> (w363:cluster{dbl[], dbl[]})  [unwired: 1 in]
          n125 = Bundle(w361, w360) -> (w362:cluster{dbl[], dbl[]})  [unwired: 1 in]
        }
        n126 = Write to Text File(file (use dialog)=w346, text=w347, error in=w344) -> (refnum out=w345:refnum<file>, error out=w343:errorcluster)  [unwired: 1 in, 1 out]
      }
    }
    n127 = Wait (ms)(milliseconds to wait=u32 1000) -> ()  [unwired: 1 out]
  }
  n128 = Unbundle(w32) -> ("System #1 Enabled/Disabled"=w31:bool, "System #2 Enabled/Disabled"=w30:bool, "System #3 Enabled/Disabled"=w29:bool)
  n129 = Close File(refnum=w41, error in=w40) -> (error out=w43:errorcluster)  [unwired: 1 out]
  n130 = case shown="True" w30 {
    tunnel: w24 -> [_ w429]
    frame False {
    }
    frame True {
      n131 = Unbundle(w429) -> ("VISA resource name out"=w428:refnum<visa-resource-name>, "error out"=w427:errorcluster)
      n132 = call <instrlib>:"Close.vi"("error in (no error)"=w427, "VISA resource name"=w428) -> ("error out"=w430:errorcluster)  [unwired: 9 in]
      n133 = call <vilib>:"Simple Error Handler.vi"("error in (no error)"=w430) -> ()  [unwired: 4 in, 5 out]
    }
  }
  n134 = case shown="True" w29 {
    tunnel: w23 -> [_ w433]
    frame False {
    }
    frame True {
      n135 = Unbundle(w433) -> ("VISA resource name out"=w431:refnum<visa-resource-name>, "error out"=w432:errorcluster)
      n136 = call <instrlib>:"Close.vi"("error in (no error)"=w432, "VISA resource name"=w431) -> ("error out"=w434:errorcluster)  [unwired: 9 in]
      n137 = call <vilib>:"Simple Error Handler.vi"("error in (no error)"=w434) -> ()  [unwired: 4 in, 5 out]
    }
  }
  n138 = call <vilib>:"Simple Error Handler.vi"("error in (no error)"=w43) -> ()  [unwired: 4 in, 5 out]
  n139 = case shown="True" w31 {
    tunnel: w25 -> [_ w437]
    frame False {
    }
    frame True {
      n140 = Unbundle(w437) -> ("VISA resource name out"=w436:refnum<visa-resource-name>, "error out"=w435:errorcluster)
      n141 = call <instrlib>:"Close.vi"("error in (no error)"=w435, "VISA resource name"=w436) -> ("error out"=w438:errorcluster)  [unwired: 9 in]
      n142 = call <vilib>:"Simple Error Handler.vi"("error in (no error)"=w438) -> ()  [unwired: 4 in, 5 out]
    }
  }
